vi "Test Log Schema Show FP.vi"(8 "error in (no error)":errorcluster, 11 "Test Info in":refnum<class "Test Info.lvclass">) -> (0 "error out":errorcluster, 2 "Schema":string, 3 "Test Info out":refnum<class "Test Info.lvclass">)   [LabVIEW 2023]
uses:
  Test Info.lvclass
  D:/eDCU LTT/VT LTT Project/Source Code/Data Analysis/Subpanel-Abstract/Subpanel-Abstract.lvclass
  C:/Program Files/National Instruments/LabVIEW 2023/vi.lib/ActorFramework/Actor/Actor.lvclass
  D:/eDCU LTT/VT LTT Project/Source Code/Data Analysis/Test Info/Test Info/Test Info.lvclass
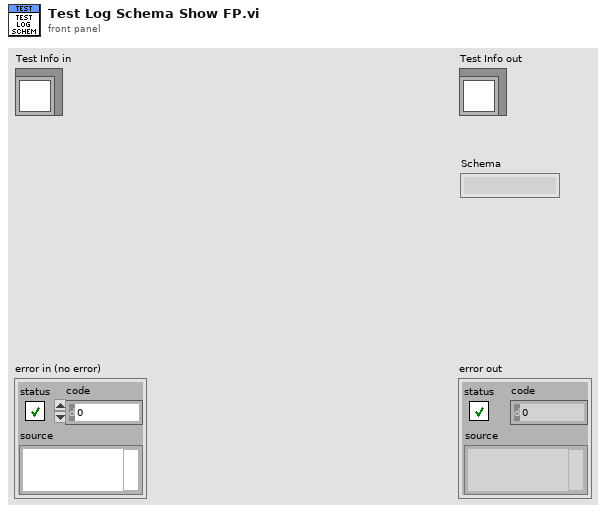
[diagram p1: front panel]
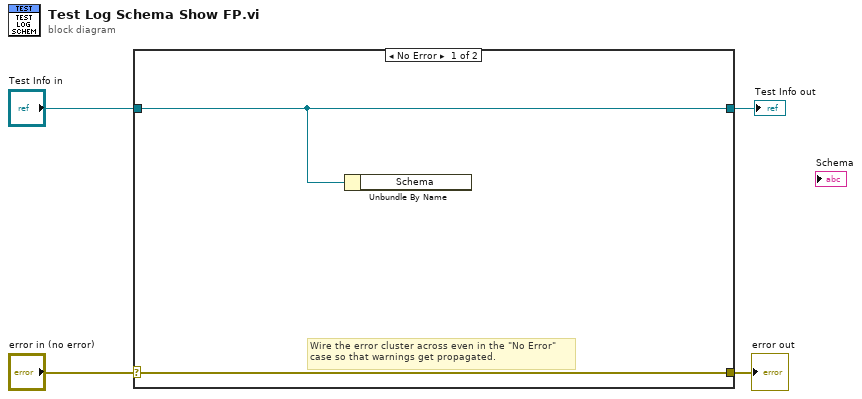
[diagram p0: block diagram]
diagram:
  n1 = case shown="No Error" "error in (no error)" {
    selector: "error in (no error)" -> [w6 w8]
    tunnel: [w6 w8] -> w3
    tunnel: [w5 w7] -> w1
    tunnel: "Test Info in" -> [w5 w7]
    frame No Error {
      # "Wire the error cluster across even in the \"No Error\"\ncase so that warnings get propagated."
      n2 = Unbundle By Name(w5) -> ()  [unwired: 1 out]
    }
    frame Error {
    }
  }
  "error out" <- w3
  "Test Info out" <- w1
